vi "Ev GoTo.vi"(8 "error in (no error)":errorcluster, 10 "Old Value":u16, 11 "LF2R IDE in":refnum<class "Main Panel.lvclass">) -> (0 "error out":errorcluster, 3 "LF2R IDE out":refnum<class "Main Panel.lvclass">)   [LabVIEW 2018, in "Main Panel.lvlib" / "Main Panel.lvclass"]
uses:
  Main Panel.lvclass
  Main Panel.lvclass/Main Panel.ctl
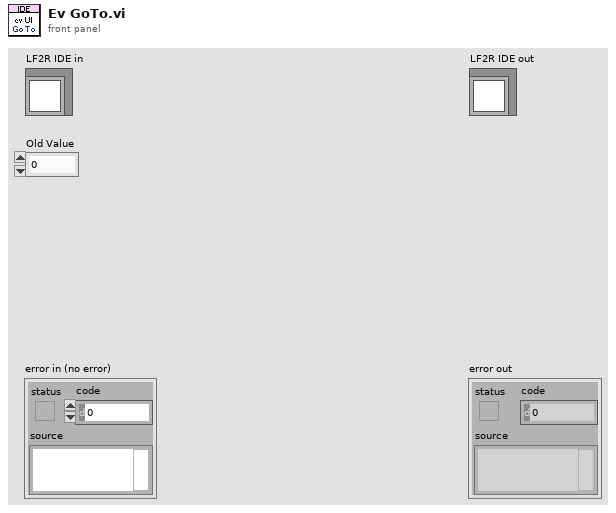
[diagram p1: front panel]
types:
  T1 = enum16{"Left Button", "Center Button", "Right Button", "Window Close"}
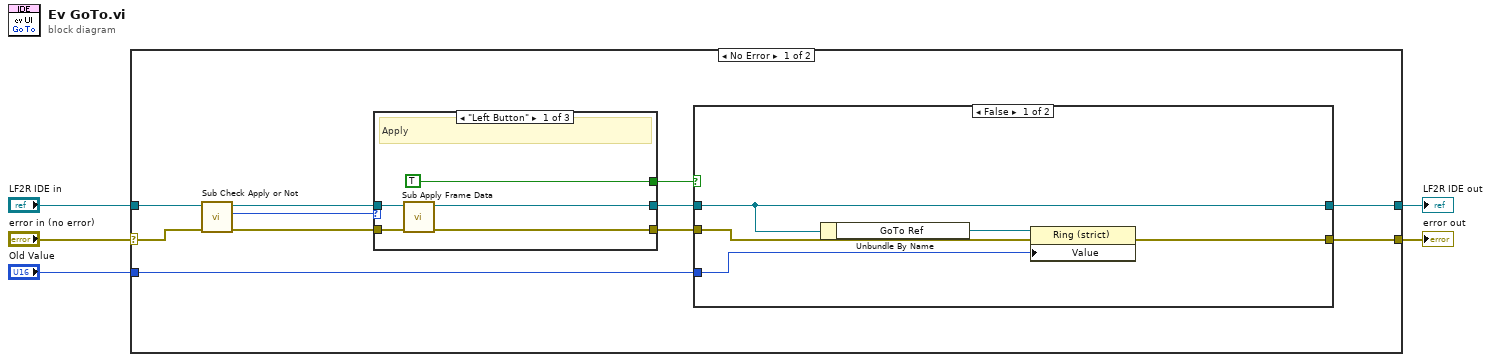
[diagram p0: block diagram]
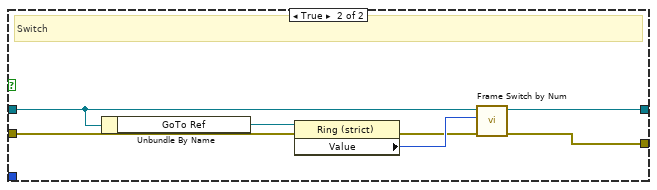
[diagram p2: hidden frame]
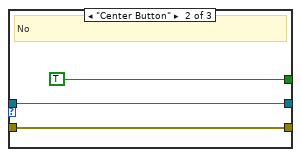
[diagram p3: hidden frame]
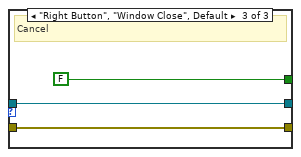
[diagram p4: hidden frame]
diagram:
  n1 = case shown="No Error" "error in (no error)" {
    selector: "error in (no error)" -> [w10 w41]
    tunnel: [w15 w41] -> w4
    tunnel: [w16 w40] -> w2
    tunnel: "LF2R IDE in" -> [w11 w40]
    tunnel: "Old Value" -> [w6 _]
    frame No Error {
      n2 = call "Sub Check Apply or Not.vi"("error in (no error)"=w10, "Main Panel in"=w11) -> ("error out"=w12:errorcluster, "Which Button?"=w14:T1, "Main Panel out"=w13:refnum<class "Main Panel.lvclass">)  [unwired: 7 in]
      n3 = case shown="\"Left Button\"" w14 {
        tunnel: w13 -> [w33 w36 w39]
        tunnel: w12 -> [w32 w35 w38]
        tunnel: [w31 w36 w39] -> w8
        tunnel: [w30 w35 w38] -> w9
        tunnel: [TRUE TRUE FALSE] -> w7
        frame "Left Button" {
          # "Apply"
          n4 = call "Sub Apply Frame Data.vi"("error in (no error)"=w32, "IDE simple in"=w33) -> ("error out"=w30:errorcluster, "IDE simple out"=w31:refnum<class "Main Panel.lvclass">)  [unwired: 8 in]
        }
        frame "Center Button" {
          # "No"
        }
        frame "Right Button", "Window Close", Default {
          # "Cancel"
        }
      }
      n5 = case shown="False" w7 {
        tunnel: [w19 w25] -> w16
        tunnel: [w18 w24] -> w15
        tunnel: w9 -> [w20 w23]
        tunnel: w8 -> [w19 w22]
        tunnel: w6 -> [w17 _]
        frame False {
          n6 = Unbundle By Name(w19) -> ("GoTo Ref"=w21:refnum<vi>)
          n7 = property class="Ring (strict)"(reference=w21, error in=w20, "Value"=w17) -> (error out=w18:errorcluster)  [unwired: 1 out]
        }
        frame True {
          # "Switch"
          n8 = Unbundle By Name(w22) -> ("GoTo Ref"=w28:refnum<vi>)
          n9 = property class="Ring (strict)"(reference=w28, error in=w23) -> (error out=w26:errorcluster, "Value"=w27:u16)  [unwired: 1 out]
          n10 = call "Frame Switch by Num.vi"("error in (no error)"=w26, "Frame Num"=w27, "LF2R IDE in"=w22) -> ("error out"=w24:errorcluster, "LF2R IDE out"=w25:refnum<class "Main Panel.lvclass">)  [unwired: 7 in]
        }
      }
    }
    frame Error {
    }
  }
  "error out" <- w4
  "LF2R IDE out" <- w2
